vi "Tokenize Tag.vi"(8 "Error In":errorcluster, 11 "Parser In":refnum<class "Parser.lvclass">) -> (0 "Error Out":errorcluster, 3 "Parser Out":refnum<class "Parser.lvclass">)   [LabVIEW 2018, in "Toolkit.lvlib" / "Parser.lvclass"]
uses:
  Parser.lvclass
  Parser.lvclass/Parser.ctl
  Tokens/EscapedVariable/EscapedVariable.lvclass
  D:/Users/cfield/Code/Field R&D Services/Mustache/trunk/src/Mustache/Public/Tokens/Public/Keyable/Keyable.lvclass
  Tokens/UnescapedVariable/UnescapedVariable.lvclass
  Tokens/BeginSection/BeginSection.lvclass
  Tokens/InvertedSection/InvertedSection.lvclass
  Tokens/EndSection/EndSection.lvclass
  Tokens/Partial/Partial.lvclass
  Tokens/Keyable/API/Keyable.lvclass
  D:/Users/cfield/Code/Field R&D Services/Mustache/trunk/src/Mustache/Public/Tokens/Public/Abstract/Abstract.lvclass
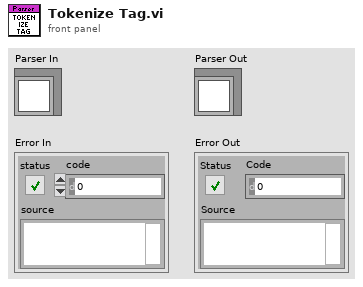
[diagram p1: front panel]
types:
  T1 = typedef "Toolkit.lvlib/Parser.lvclass/Tag Types.ctl" = enum16{"Escaped Variable", "{} Unescaped Variable", "& Unescaped Variable", "Begin Section", "Inverted Section", "End Section", "Comment", "Partial", "Set Delimiter"}
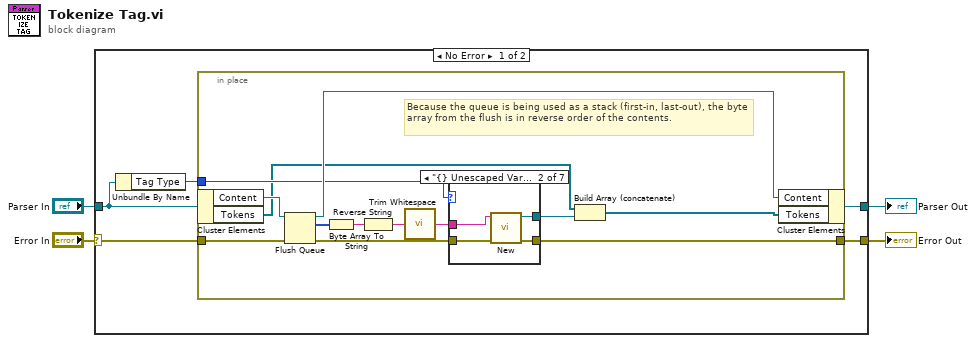
[diagram p0: block diagram]
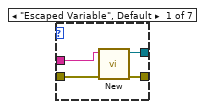
[diagram p2: hidden frame]
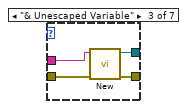
[diagram p3: hidden frame]
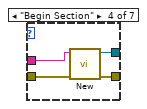
[diagram p4: hidden frame]
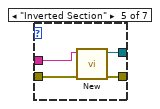
[diagram p5: hidden frame]
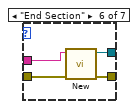
[diagram p6: hidden frame]
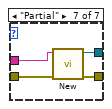
[diagram p7: hidden frame]
diagram:
  n1 = case shown="No Error" "Error In" {
    selector: "Error In" -> [w7 w51]
    tunnel: [w9 w51] -> w4
    tunnel: [w8 w52] -> w3
    tunnel: "Parser In" -> [w6 w52]
    frame No Error {
      n2 = Unbundle By Name(w6) -> ("Tag Type"=w5:T1)
      n3 = in-place {
        in-place-border: [w15] -> w9
        in-place-border: w7 -> [w19]
        in-place-border: w5 -> [w13]
        # "Because the queue is being used as a stack (first-in, last-out), the byte array from the flush is in reverse order of the contents."
        n4 = in-place-cluster #1(w6) -> ("Content"=w22:refnum<queue>, "Tokens"=w12:refnum<class "Abstract.lvclass">[])
        n5 = Flush Queue(queue=w22, error in (no error)=w19) -> (queue out=w21:refnum<queue>, remaining elements=w20:u8[], error out=w16:errorcluster)
        n6 = Byte Array To String(unsigned byte array=w20) -> (string=w18:string)
        n7 = Reverse String(1:w18) -> (0:w17:string)
        n8 = call <vilib>:"Trim Whitespace.vi"("string"=w17) -> ("trimmed string"=w14:string)  [unwired: 1 in]
        n9 = case shown="\"{} Unescaped Variable\"" w13 {
          tunnel: w16 -> [w26 w29 w33 w37 w41 w45 w49]
          tunnel: [w25 w28 w32 w36 w40 w44 w48] -> w15
          tunnel: w14 -> [w24 w30 w34 w38 w42 w46 w50]
          tunnel: [w23 w27 w31 w35 w39 w43 w47] -> w11
          frame "Escaped Variable", Default {
            n10 = call "New.vi"("Error In"=w26, "Key"=w24) -> ("Error Out"=w25:errorcluster, "Escaped Variable"=w23:refnum<class "EscapedVariable.lvclass">)  [unwired: 8 in]
          }
          frame "{} Unescaped Variable" {
            n11 = call "New.vi"("Error In"=w29, "Key"=w30) -> ("Error Out"=w28:errorcluster, "Unescaped Variable"=w27:refnum<class "UnescapedVariable.lvclass">)  [unwired: 8 in]
          }
          frame "& Unescaped Variable" {
            n12 = call "New.vi"("Error In"=w33, "Key"=w34) -> ("Error Out"=w32:errorcluster, "Unescaped Variable"=w31:refnum<class "UnescapedVariable.lvclass">)  [unwired: 8 in]
          }
          frame "Begin Section" {
            n13 = call "New.vi"("Error In"=w37, "Key"=w38) -> ("Error Out"=w36:errorcluster, "Begin Section"=w35:refnum<class "BeginSection.lvclass">)  [unwired: 8 in]
          }
          frame "Inverted Section" {
            n14 = call "New.vi"("Error In"=w41, "Key"=w42) -> ("Error Out"=w40:errorcluster, "Inverted Section"=w39:refnum<class "InvertedSection.lvclass">)  [unwired: 8 in]
          }
          frame "End Section" {
            n15 = call "New.vi"("Error In"=w45, "Key"=w46) -> ("Error Out"=w44:errorcluster, "End Section"=w43:refnum<class "EndSection.lvclass">)  [unwired: 8 in]
          }
          frame "Partial" {
            n16 = call "New.vi"("Error In"=w49, "Key"=w50) -> ("Error Out"=w48:errorcluster, "Partial"=w47:refnum<class "Partial.lvclass">)  [unwired: 8 in]
          }
        }
        n17 = Build Array (concatenate)(w12, w11) -> (w10:refnum<class "Abstract.lvclass">[])
        n18 = in-place-cluster #1("Content"=w21, "Tokens"=w10) -> (w8:refnum<class "Parser.lvclass">)
      }
    }
    frame Error {
    }
  }
  "Error Out" <- w4
  "Parser Out" <- w3
